vi "clear Session Data.vi"(0 "Session in":refnum<class "SequenceFile.lvclass">, 11 "error in":errorcluster) -> (4 "Session out":refnum<class "SequenceFile.lvclass">, 15 "error out":errorcluster)   [LabVIEW 2020, in "TSS.lvlib" / "SequenceFile.lvclass"]
uses:
  SequenceFile.lvclass
  SequenceFile.lvclass/SequenceFile.ctl
  <userlib>/_Session Fwk/Session - Root.lvclass
  Engine/Engine.lvclass
  VariableContainer/VariableContainer.lvclass
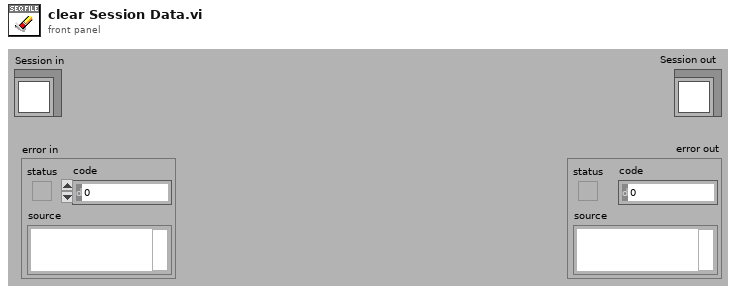
[diagram p1: front panel]
types:
  T1 = typedef "TSS.lvlib/VariableContainer.lvclass/Session Handle.ctl" = refnum<data-value>
  T2 = typedef "TSS.lvlib/Engine.lvclass/Session Handle.ctl" = refnum<data-value>
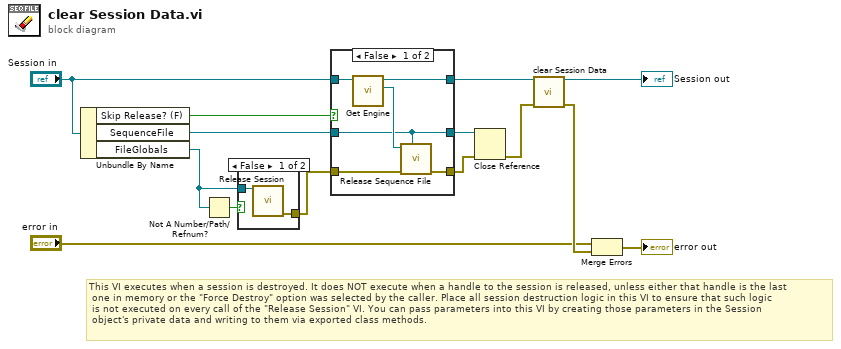
[diagram p0: block diagram]
diagram:
  # "This VI executes when a session is destroyed. It does NOT execute when a handle to the session is released, unless either that handle is the last\n one in memory or the \"Force Destroy\" option was selected by the caller. Place all session destruction logic in this VI to ensure that such logic\n is not executed on every call of the \"Release Session\" VI. You can pass parameters into this VI by creating those parameters in the Session \n object's private data and writing to them via exported class methods."
  n1 = Unbundle By Name("Session in") -> ("Skip Release? (F)"=w1:bool, "SequenceFile"=w11:refnum<k7>, "FileGlobals"=w7:T1)
  n2 = Not A Number/Path/Refnum?(number/path/refnum=w7) -> (NaN/Path/Refnum?=w6:bool)
  n3 = case shown="False" w6 {
    tunnel: w7 -> [w16 _]
    tunnel: [w15 _] -> w5
    frame False {
      n4 = call "Release Session.vi"("Session Handle"=w16) -> ("error out"=w15:errorcluster)  [unwired: 14 in]
    }
    frame True {
    }
  }
  n5 = case shown="False" w1 {
    tunnel: [w22 w23] -> w12
    tunnel: w11 -> [w17 w24]
    tunnel: w5 -> [w21 w23]
    tunnel: "Session in" -> [w20 w25]
    tunnel: [w19 w25] -> w3
    tunnel: [w17 w24] -> w2
    frame False {
      n6 = call "Get Engine.vi"("SequenceFile in"=w20) -> ("Engine"=w18:T2, "SequenceFile out"=w19:refnum<class "SequenceFile.lvclass">)  [unwired: 8 in, 1 out]
      n7 = call "Release Sequence File.vi"("SequenceFile"=w17, "error in (no error)"=w21, "Session Handle in"=w18) -> ("error out"=w22:errorcluster)  [unwired: 7 in, 1 out]
    }
    frame True {
    }
  }
  n8 = Close Reference(reference=w2, error in (no error)=w12) -> (error out=w10:errorcluster)
  n9 = call-parent "clear Session Data.vi"("OBJ - Measurement Session in"=w3, "error in"=w10) -> ("OBJ - Measurement Session out"=→"Session out":refnum<class "SequenceFile.lvclass">, "error out"=w13:errorcluster)  [unwired: 12 in]
  n10 = Merge Errors("error in", w13) -> (→"error out":errorcluster)
